vi "LoadUDPAddress.vi"(8 "error in (no error)":errorcluster, 11 "TrigBoxINIFileClass in":refnum<class "TrigBoxINIFileClass.lvclass">) -> (0 "error out":errorcluster, 2 "UPDAddress":string, 3 "TrigBoxINIFileClass out":refnum<class "TrigBoxINIFileClass.lvclass">)   [LabVIEW 2013, in "TrigBoxINIFileClass.lvclass"]
uses:
  TrigBoxINIFileClass.lvclass
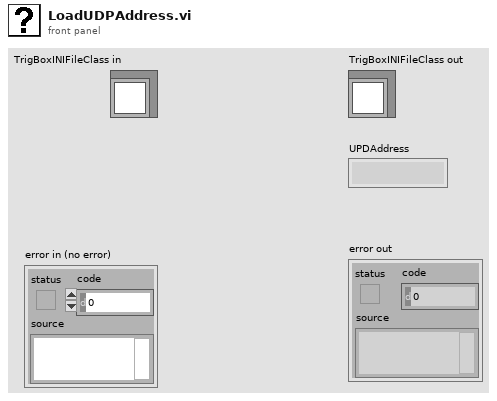
[diagram p1: front panel]
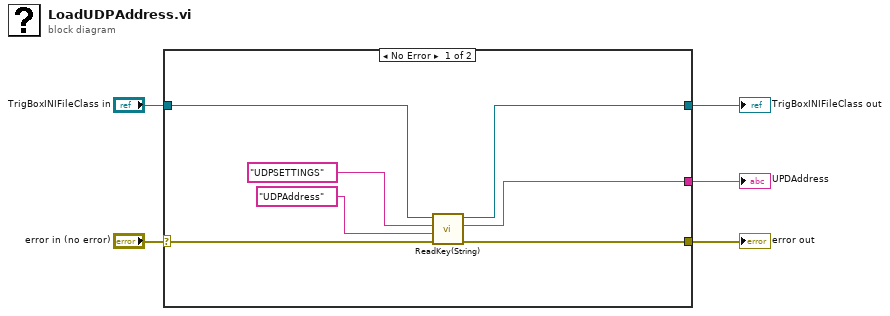
[diagram p0: block diagram]
diagram:
  n1 = case shown="No Error" "error in (no error)" {
    selector: "error in (no error)" -> [w12 w14]
    tunnel: [w8 w14] -> w4
    tunnel: [w7 w13] -> w2
    tunnel: "TrigBoxINIFileClass in" -> [w11 w13]
    tunnel: [w6 _] -> w1
    frame No Error {
      n2 = call-dynamic "ReadKey(String).vi"("error in"=w12, "key"="UDPAddress" ("section"), "section"="UDPSETTINGS", "INIFileClass in"=w11) -> ("error out"=w8:errorcluster, "StringOut"=w6:string, "INIFileClass out"=w7:refnum<class "TrigBoxINIFileClass.lvclass">)  [unwired: 5 in]
    }
    frame Error {
    }
  }
  "error out" <- w4
  "TrigBoxINIFileClass out" <- w2
  "UPDAddress" <- w1
